vi "RunOperation.vi"(10 "Inputs":string[](array[string]), 11 "MassCompile in":refnum<class "MassCompile.lvclass">) -> (1 "Output/Failure":string, 2 "CLI Process Return Code":i32, 3 "MassCompile out":refnum<class "MassCompile.lvclass">)   [LabVIEW 2014, in "MassCompile.lvclass"]
uses:
  MassCompile.lvclass
  MassCompile.lvclass/MassCompile.ctl
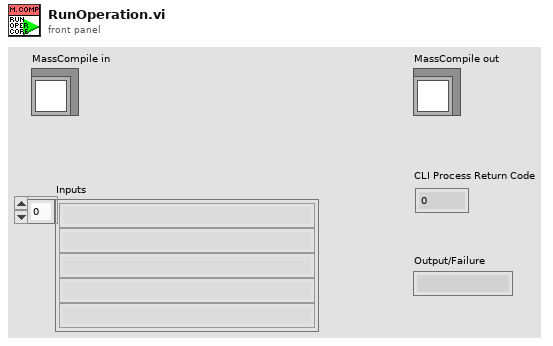
[diagram p1: front panel]
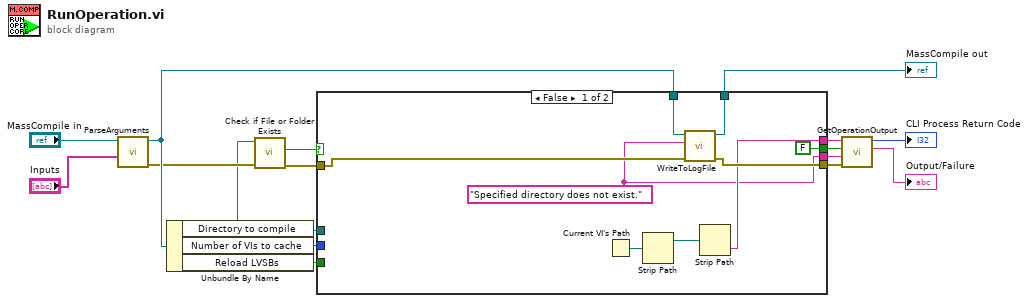
[diagram p0: block diagram]
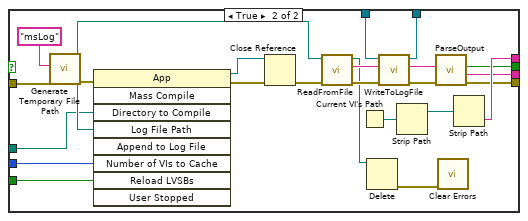
[diagram p2: hidden frame]
diagram:
  n1 = call "ParseArguments.vi"("Inputs"="Inputs", "MassCompile in"="MassCompile in") -> ("error out"=w4:errorcluster, "MassCompile out"=w8:refnum<class "MassCompile.lvclass">)  [unwired: 8 in]
  n2 = Unbundle By Name(w8) -> ("Directory to compile"=w2:path, "Number of VIs to cache"=w10:u32, "Reload LVSBs"=w9:bool)
  n3 = call <vilib>:"Check if File or Folder Exists.vi"("error in (no error)"=w4, "path"=w2) -> ("error out"=w3:errorcluster, "file or folder exists?"=w1:bool)  [unwired: 7 in, 1 out]
  n4 = case shown="False" w1 {
    tunnel: [w19 w45] -> w15
    tunnel: [FALSE ("Is successful?") w44] -> w14
    tunnel: [w17 w43] -> w13
    tunnel: w10 -> [_ w42]
    tunnel: w9 -> [_ w41]
    tunnel: w8 -> [w25 w38]
    tunnel: [w22 w37] -> w7
    tunnel: [w23 w34] -> w6
    tunnel: w3 -> [w24 w27]
    tunnel: w2 -> [_ w26]
    frame False {
      w17 = "Specified directory does not exist." ("File content in")
      n5 = Current VI's Path() -> (path=w21:path)
      n6 = Strip Path(path=w21) -> (stripped path=w20:path)  [unwired: 1 out]
      n7 = call "WriteToLogFile.vi"("error in"=w24, "File content in"=w17, "MassCompile in"=w25) -> ("error out"=w23:errorcluster, "MassCompile out"=w22:refnum<class "MassCompile.lvclass">)  [unwired: 6 in, 1 out]
      n8 = Strip Path(path=w20) -> (name=w19:string)  [unwired: 1 out]
    }
    frame True {
      n9 = call <vilib>:"Generate Temporary File Path.vi"("error in (no error)"=w27, "Temporary File Extension (tmp)"="msLog") -> ("error out"=w28:errorcluster, "Unique Temporary File Path"=w36:path)  [unwired: 8 in]
      n10 = invoke class="App" method="Mass Compile"(error in=w28, "Directory to Compile"=w26, "Log File Path"=w36, "Number of VIs to Cache"=w42, "Reload LVSBs"=w41) -> (reference out=w49:refnum<vi>, error out=w48:errorcluster)  [unwired: 4 in, 7 out]
      n11 = Close Reference(reference=w49, error in (no error)=w48) -> (error out=w39:errorcluster)
      n12 = call "ReadFromFile.vi"("error in (no error)"=w39, "Temporary File Path in"=w36) -> ("error out"=w35:errorcluster, "File content"=w33:string, "Temporary File Path out"=w30:path)  [unwired: 7 in]
      n13 = Current VI's Path() -> (path=w47:path)
      n14 = Delete(path (use dialog)=w30) -> (error out=w32:errorcluster)  [unwired: 4 in, 2 out]
      n15 = call "WriteToLogFile.vi"("error in"=w35, "File content in"=w33, "MassCompile in"=w38) -> ("error out"=w31:errorcluster, "File content out"=w29:string, "MassCompile out"=w37:refnum<class "MassCompile.lvclass">)  [unwired: 6 in]
      n16 = Strip Path(path=w47) -> (stripped path=w46:path)  [unwired: 1 out]
      n17 = call "ParseOutput.vi"("error in (no error)"=w31, "File content"=w29) -> ("error out"=w34:errorcluster, "Mass compile output"=w43:string, "Is successful?"=w44:bool)  [unwired: 7 in]
      n18 = call <vilib>:"Clear Errors.vi"("error in (no error)"=w32) -> ()  [unwired: 5 in, 2 out]
      n19 = Strip Path(path=w46) -> (name=w45:string)  [unwired: 1 out]
    }
  }
  "MassCompile out" <- w7
  n20 = call "GetOperationOutput.vi"("error in (no error)"=w6, "Operation Output/Error In"=w13, "Operation succeeded?"=w14, "Operation Name"=w15) -> ("Operation Output/Error Out"=→"Output/Failure":string, "CLI Process Return Code"=→"CLI Process Return Code":i32)  [unwired: 6 in]
